vi "ReMiRCDelta put obiect.vi"(7 "move to":T1(ring), 8 "error in (no error)":errorcluster, 10 "off setY":dbl, 11 "off setX":dbl) -> (0 "error in (no error) 2":errorcluster)   [LabVIEW 2019]
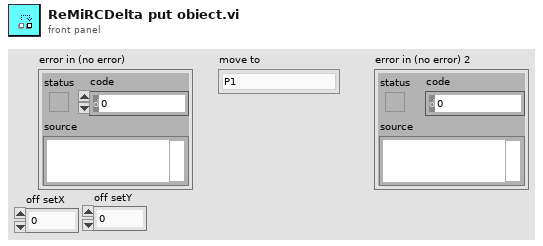
[diagram p1: front panel]
types:
  T1 = enum16{"P1", "P2", "P3", "P4", "P5", "P6", "OUT", "take a picture"}
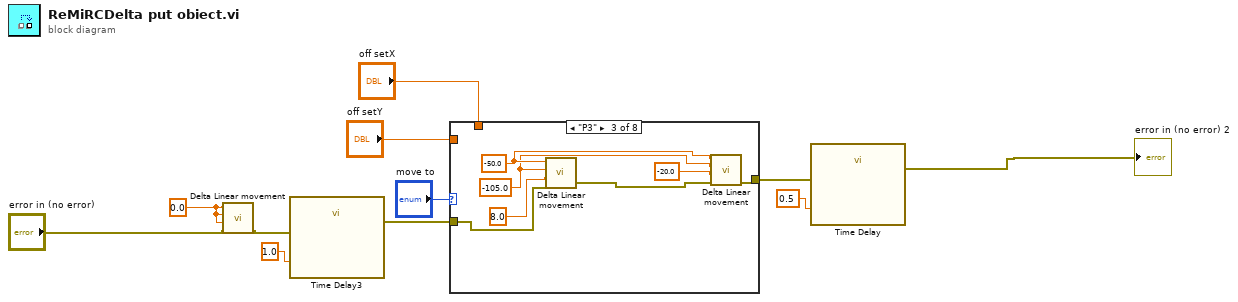
[diagram p0: block diagram]
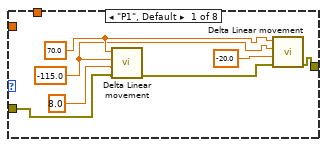
[diagram p2: hidden frame]
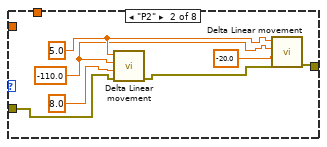
[diagram p3: hidden frame]
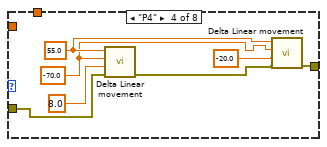
[diagram p4: hidden frame]
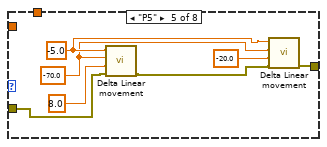
[diagram p5: hidden frame]
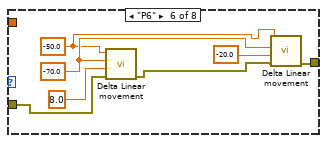
[diagram p6: hidden frame]
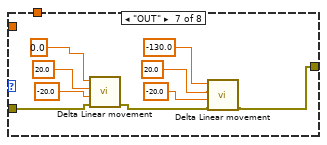
[diagram p7: hidden frame]
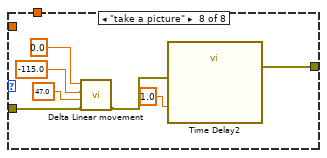
[diagram p8: hidden frame]
diagram:
  w4 = 0.0 ("x0")
  n1 = call "Delta Linear movement.vi"("error in (no error)"="error in (no error)", "z0"=w4, "y0"=w4, "x0"=w4) -> ("error out"=w2:errorcluster)  [unwired: 7 in]
  n2 = call "Time Delay3"("error in (no error)"=w2, "Delay Time (s)"=1.0 ("x0")) -> ("error out"=w7:errorcluster)  [unwired: 9 in]
  n3 = case shown="\"P3\"" "move to" {
    tunnel: w7 -> [w18 w25 w32 w39 w46 w53 w62 w64]
    tunnel: [w13 w19 w26 w36 w40 w50 w54 w68] -> w10
    tunnel: "off setX" -> [_ _ _ _ _ _ _ _]
    tunnel: "off setY" -> [_ _ _ _ _ _ _ _]
    frame "P1", Default {
      w15 = -115.0 ("y0")
      w16 = 70.0 ("x0")
      n4 = call "Delta Linear movement.vi"("error in (no error)"=w18, "z0"=8.0, "y0"=w15, "x0"=w16) -> ("error out"=w12:errorcluster)  [unwired: 7 in]
      n5 = call "Delta Linear movement.vi"("error in (no error)"=w12, "z0"=-20.0, "y0"=w15, "x0"=w16) -> ("error out"=w13:errorcluster)  [unwired: 7 in]
    }
    frame "P2" {
      w22 = -110.0 ("y0")
      w23 = 5.0 ("x0")
      n6 = call "Delta Linear movement.vi"("error in (no error)"=w25, "z0"=8.0, "y0"=w22, "x0"=w23) -> ("error out"=w20:errorcluster)  [unwired: 7 in]
      n7 = call "Delta Linear movement.vi"("error in (no error)"=w20, "z0"=-20.0, "y0"=w22, "x0"=w23) -> ("error out"=w19:errorcluster)  [unwired: 7 in]
    }
    frame "P3" {
      w29 = -105.0 ("y0")
      w30 = -50.0 ("x0")
      n8 = call "Delta Linear movement.vi"("error in (no error)"=w32, "z0"=8.0, "y0"=w29, "x0"=w30) -> ("error out"=w27:errorcluster)  [unwired: 7 in]
      n9 = call "Delta Linear movement.vi"("error in (no error)"=w27, "z0"=-20.0, "y0"=w29, "x0"=w30) -> ("error out"=w26:errorcluster)  [unwired: 7 in]
    }
    frame "P4" {
      w34 = -70.0 ("y0")
      w35 = 55.0 ("x0")
      n10 = call "Delta Linear movement.vi"("error in (no error)"=w39, "z0"=8.0, "y0"=w34, "x0"=w35) -> ("error out"=w37:errorcluster)  [unwired: 7 in]
      n11 = call "Delta Linear movement.vi"("error in (no error)"=w37, "z0"=-20.0, "y0"=w34, "x0"=w35) -> ("error out"=w36:errorcluster)  [unwired: 7 in]
    }
    frame "P5" {
      w43 = -70.0 ("y0")
      w44 = -5.0 ("x0")
      n12 = call "Delta Linear movement.vi"("error in (no error)"=w46, "z0"=8.0, "y0"=w43, "x0"=w44) -> ("error out"=w41:errorcluster)  [unwired: 7 in]
      n13 = call "Delta Linear movement.vi"("error in (no error)"=w41, "z0"=-20.0, "y0"=w43, "x0"=w44) -> ("error out"=w40:errorcluster)  [unwired: 7 in]
    }
    frame "P6" {
      w48 = -70.0 ("y0")
      w47 = -50.0 ("x0")
      n14 = call "Delta Linear movement.vi"("error in (no error)"=w53, "z0"=8.0, "y0"=w48, "x0"=w47) -> ("error out"=w51:errorcluster)  [unwired: 7 in]
      n15 = call "Delta Linear movement.vi"("error in (no error)"=w51, "z0"=-20.0, "y0"=w48, "x0"=w47) -> ("error out"=w50:errorcluster)  [unwired: 7 in]
    }
    frame "OUT" {
      n16 = call "Delta Linear movement.vi"("error in (no error)"=w62, "z0"=-20.0, "y0"=20.0, "x0"=0.0) -> ("error out"=w58:errorcluster)  [unwired: 7 in]
      n17 = call "Delta Linear movement.vi"("error in (no error)"=w58, "z0"=-20.0, "y0"=20.0, "x0"=-130.0) -> ("error out"=w54:errorcluster)  [unwired: 7 in]
    }
    frame "take a picture" {
      n18 = call "Delta Linear movement.vi"("error in (no error)"=w64, "z0"=47.0, "y0"=-115.0, "x0"=0.0) -> ("error out"=w63:errorcluster)  [unwired: 7 in]
      n19 = call "Time Delay2"("error in (no error)"=w63, "Delay Time (s)"=1.0) -> ("error out"=w68:errorcluster)  [unwired: 9 in]
    }
  }
  n20 = call "Time Delay"("error in (no error)"=w10, "Delay Time (s)"=0.5) -> ("error out"=→"error in (no error) 2":errorcluster)  [unwired: 9 in]
